vi "Read Tag Name.vi"(8 "error in (no error)":errorcluster, 11 "IPersist in":refnum<class "IPersist.lvclass">) -> (0 "error out":errorcluster, 2 "Tag Name":string, 3 "IPersist out":refnum<class "IPersist.lvclass">)   [LabVIEW 2019, in "IPersist.lvlib" / "IPersist.lvclass"]
uses:
  <vilib>/gpm_packages/@cs/persistence/source/IPersist/IPersist.lvclass
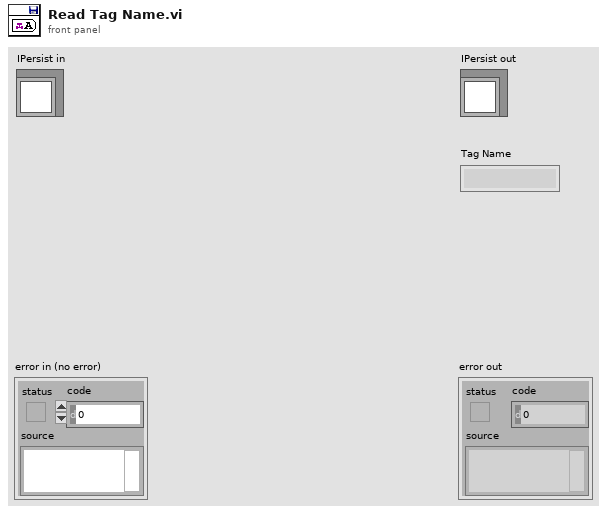
[diagram p1: front panel]
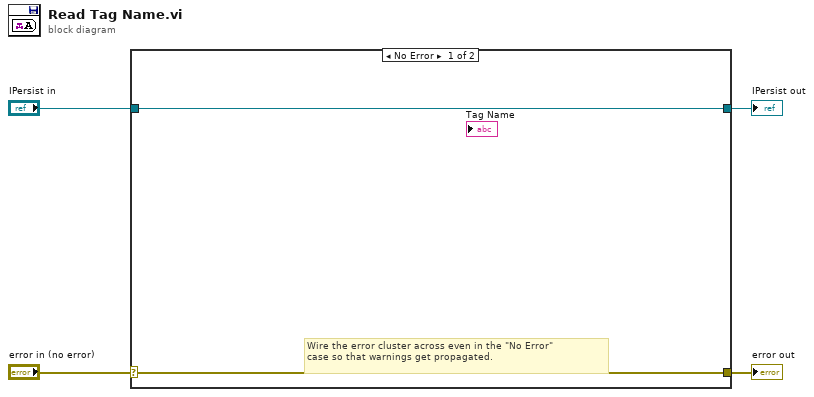
[diagram p0: block diagram]
diagram:
  n1 = case shown="No Error" "error in (no error)" {
    selector: "error in (no error)" -> [w5 w8]
    tunnel: [w5 w8] -> w3
    tunnel: [w6 w7] -> w1
    tunnel: "IPersist in" -> [w6 w7]
    frame No Error {
      # "Wire the error cluster across even in the \"No Error\"\ncase so that warnings get propagated."
    }
    frame Error {
    }
  }
  "error out" <- w3
  "IPersist out" <- w1
